vi "压力损失.vi"(0 "压力损失":sgl, 1 "压力损失判定条件":cluster{"下限":dbl, "上限":dbl}, 3 "错误输入":errorcluster) -> (8 "OK":bool, 10 "错误输出":errorcluster)   [LabVIEW 2017]
uses:
  Global_Variable/Global.vi
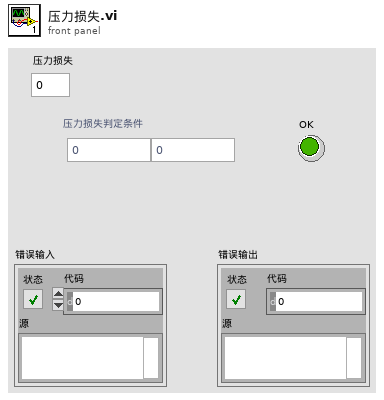
[diagram p1: front panel]
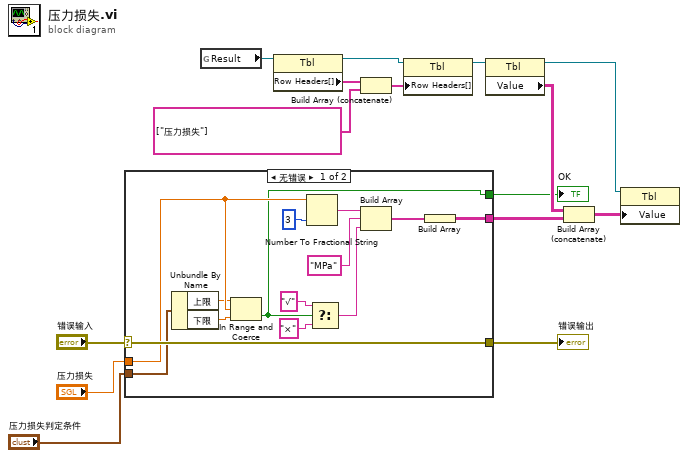
[diagram p0: block diagram]
diagram:
  n1 = case shown="无错误" "错误输入" {
    selector: "错误输入" -> [w21 w30]
    tunnel: [w21 w30] -> w14
    tunnel: [w23 _] -> w5
    tunnel: "压力损失判定条件" -> [w20 _]
    tunnel: "压力损失" -> [w19 _]
    tunnel: [w16 _] -> w1
    frame No Error {
      n2 = Unbundle By Name(w20) -> ("上限"=w18:dbl, "下限"=w17:dbl)
      n3 = In Range and Coerce(upper limit=w18, x=w19, lower limit=w17) -> (In Range?=w16:bool)  [unwired: 1 out]
      n4 = Number To Fractional String(number=w19, precision (6)=i16 3 ("精度(6)")) -> (F-format string=w28:string)  [unwired: 2 in]
      n5 = Select(t="√", s=w16, f="×") -> (s? t:f=w24:string)
      n6 = Build Array(w28, "MPa" ("元素"), w24) -> (w22:string[])
      n7 = Build Array(w22) -> (w23:string[][])
    }
    frame Error {
    }
  }
  "错误输出" <- w14
  "OK" <- w1
  n8 = global read "Global.vi" "Result"() -> (w13:refnum<vi>)
  n9 = property class="Tbl"(reference=w13) -> (reference out=w9:refnum<vi>, "Row Headers[]"=w12:string[])  [unwired: 1 in, 1 out]
  n10 = Build Array (concatenate)(w12, string[] ["压力损失"] ("元素")) -> (w10:string[])
  n11 = property class="Tbl"(reference=w9, "Row Headers[]"=w10) -> (reference out=w8:refnum<vi>)  [unwired: 1 in, 1 out]
  n12 = property class="Tbl"(reference=w8) -> (reference out=w7:refnum<vi>, "Value"=w6:string[][])  [unwired: 1 in, 1 out]
  n13 = Build Array (concatenate)(w6, w5) -> (w4:string[][])
  n14 = property class="Tbl"(reference=w7, "Value"=w4) -> ()  [unwired: 1 in, 2 out]
